vi "Update_Data_Packet_From_Processed_Bytes.vi"(8 "error in (no error)":errorcluster, 11 "Processed Bytes":u8[](array[numeric])) -> (0 "error out":errorcluster)   [LabVIEW 2017]
uses:
  Controls/Packet/Packet_Type.ctl
  Controls/Data Packets/Data_Packet_FGV_Commands.ctl
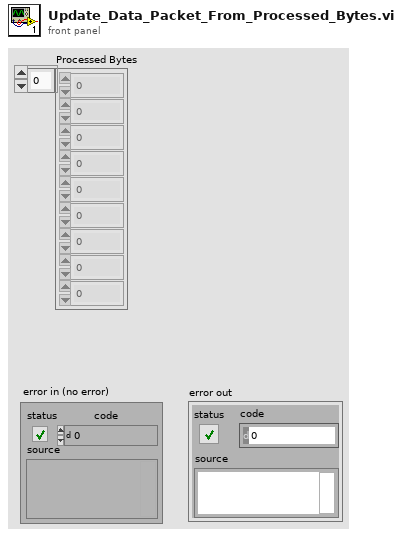
[diagram p1: front panel]
types:
  T1 = typedef "Packet_Type.ctl" = enum16{"Data", "Connection Management", "Remote Request", "Error/Status"}
  T2 = typedef "Packet_Priority.ctl" = enum16{"LOW", "HIGH"}
  T3 = typedef "Data_Packet_FGV_Commands.ctl" = enum16{"Update Packet", "Load", "Read Packet Parameters", "Write Packet Parameters", "Read Packet Parameter", "Write Packet Parameter", "Read Data Packets", "Read Data Packet", "Read Data Packet by Parameter Name", "Get Parameter Node and Frame ID", "Read Data Packet from Node ID and Frame ID"}
  T4 = typedef "Data_Packet.ctl" = cluster{"Packet":T5, "Parameters":T7[], "Last Received Time (ms)":u64, "Receive count":u32, "Transmit count":u32, "Transmit interval (ms)":u32, "Last Transmitted Time (ms)":u64, "Receive interval (ms)":u32}
  T5 = typedef "Packet.ctl" = cluster{"Raw Bytes":u8[], "Checksum":bool, "Direction":T6, "Processed Bytes":u8[], "Node ID":u8, "Packet type":T1, "Frame Data":u32, "Priority":T2, "Frame ID":u8}
  T6 = typedef "Packet_Direction.ctl" = enum16{"Transmit", "Receive", "Bidirectional"}
  T7 = typedef "Parameter.ctl" = cluster{"Parameter name":string, "Node name":string, "Node ID":u8, "Frame name":string, "Frame ID":u8, "Data type":T8, "Start Bit":i32, "Bit Length":i32, "Factor":dbl, "Offset":dbl, "Minimum":dbl, "Maximum":dbl, "Descriptor":string, "Enum values":string[], "Value":string}
  T8 = typedef "Parameter_Data_Type.ctl" = enum16{"BOOL", "UNSIGNED", "SIGNED", "FLOAT32", "ENUM"}
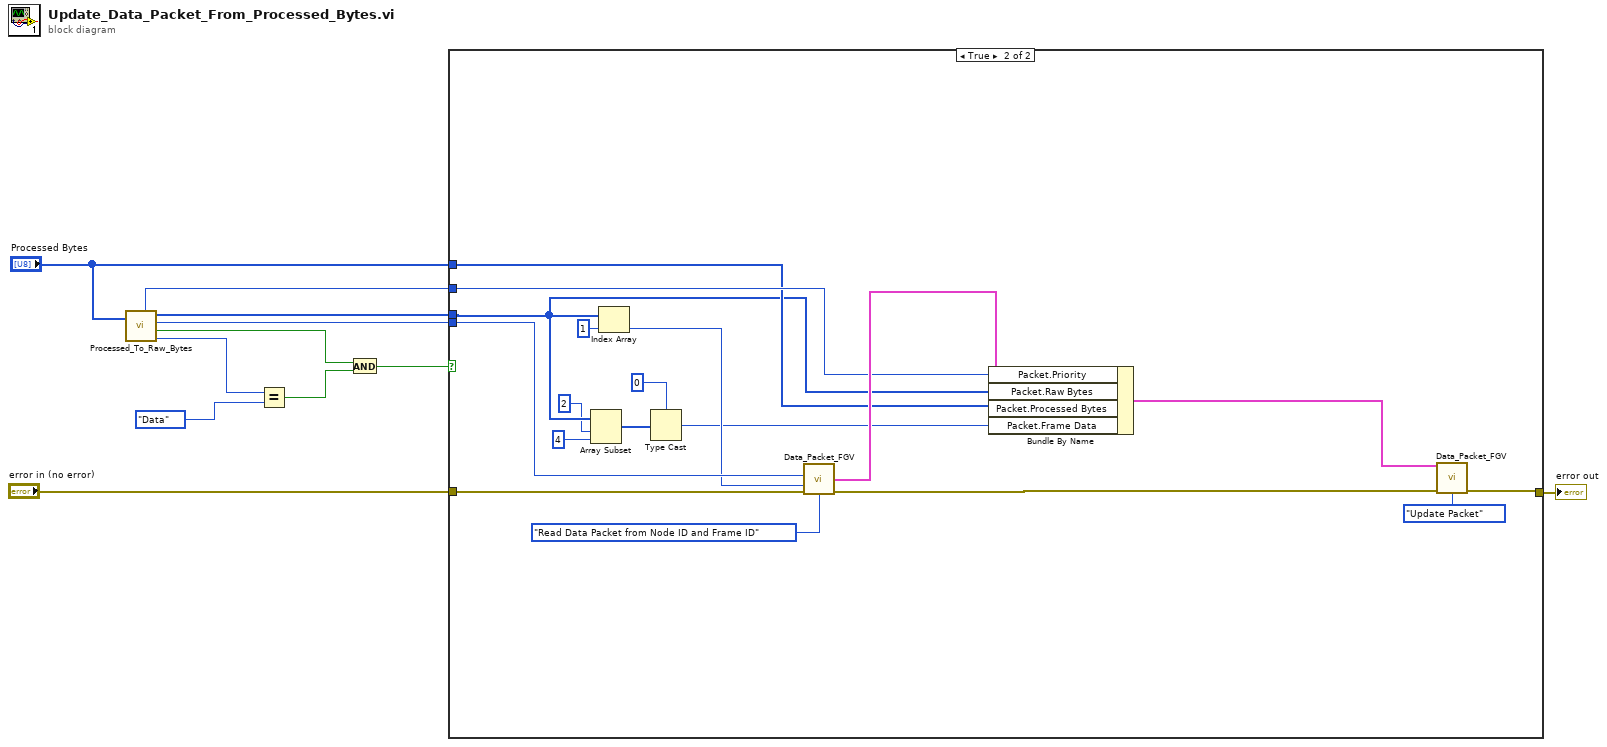
[diagram p0: block diagram]
diagram:
  n1 = call "Processed_To_Raw_Bytes.vi"("Processed Bytes"="Processed Bytes") -> ("Packet Type"=w10:T1, "Checksum"=w4:bool, "Node ID"=w8:u8, "Raw Bytes"=w7:u8[], "Priority"=w5:T2)  [unwired: 1 in]
  n2 = Equal?(x=w10, y=Packet_Type."Data") -> (x = y?=w3:bool)
  n3 = And(x=w4, y=w3) -> (x .and. y?=w2:bool)
  n4 = case shown="True" w2 {
    tunnel: "error in (no error)" -> [w12 w29]
    tunnel: w8 -> [_ w28]
    tunnel: w7 -> [_ w22]
    tunnel: "Processed Bytes" -> [_ w23]
    tunnel: w5 -> [_ w24]
    tunnel: [w12 w13] -> w1
    frame False {
    }
    frame True {
      n5 = Array Subset(array=w22, index=2, length=4) -> (w19:u8[])
      n6 = Index Array(array=w22, index=1) -> (element=w26:u8)
      n7 = Type Cast(type=u32 0, x=w19) -> (*(type *) &x=w17:u32)
      n8 = call "Data_Packet_FGV.vi"("Node ID"=w28, "Frame ID"=w26, "error in (no error)"=w29, "Commands"=Data_Packet_FGV_Commands."Read Data Packet from Node ID and Frame ID") -> ("Data_Packet Out"=w25:T4, "error out"=w16:errorcluster)  [unwired: 6 in, 4 out]
      n9 = Bundle By Name(cluster=w25, "Packet.Priority"=w24, "Packet.Raw Bytes"=w22, "Packet.Processed Bytes"=w23, "Packet.Frame Data"=w17) -> (w15:T4)
      n10 = call "Data_Packet_FGV.vi"("Data_Packet In"=w15, "error in (no error)"=w16, "Commands"=Data_Packet_FGV_Commands."Update Packet") -> ("error out"=w13:errorcluster)  [unwired: 7 in, 5 out]
    }
  }
  "error out" <- w1
